vi "Caraya Time Measurement.vi"() -> (2 "Caraya report":string, 3 "ICov Testing time (seconds)":dbl)   [LabVIEW 2018]
panel:
  # "Caraya"
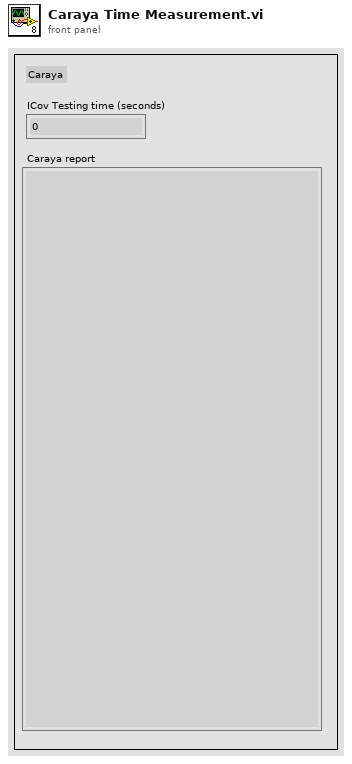
[diagram p1: front panel]
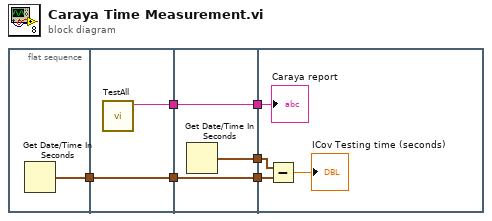
[diagram p0: block diagram]
diagram:
  n1 = flat-sequence {
    tunnel: [w7] -> w6
    tunnel: [w9] -> w5
    tunnel: w6 -> [w9]
    tunnel: [w8] -> w1
    tunnel: [w12] -> w4
    tunnel: [w11] -> w3
    tunnel: w5 -> [w11]
    tunnel: [w10] -> w2
    tunnel: w1 -> [w10]
    tunnel: w4 -> [w14]
    tunnel: w3 -> [w15]
    tunnel: w2 -> [w13]
    frame #0 {
      n2 = Get Date/Time In Seconds() -> (seconds since 1Jan1904=w7:timestamp)
    }
    frame #1 {
      n3 = call "TestAll.vi"() -> ("report"=w8:string)  [unwired: 10 in, 1 out]
    }
    frame #2 {
      n4 = Get Date/Time In Seconds() -> (seconds since 1Jan1904=w12:timestamp)
    }
    frame #3 {
      n5 = Subtract(x=w14, y=w15) -> (x-y=→"ICov Testing time (seconds)":dbl)
      "Caraya report" <- w13
    }
  }
